vi "LVClasse_Phase GetStatisticDatas.vi"(0 "Phase in":refnum<class "Phase.lvclass">, 11 "error in (no error)":errorcluster) -> (4 "Phase out":refnum<class "Phase.lvclass">, 6 "StatisticsData":T1, 15 "error out":errorcluster)   [LabVIEW 2020, in "Phase.lvclass"]
doc: "Phase statistic data getter.\n\n--------------------------------------------------------------------------------\n\n<B>PhaseIn </B> : Phase object.\n<B>PhaseOut </B> : Phase object.\n<B>rms </B> : Phase root mean square deviation.\n<B>pv </B> : Phase peak to valley.\n<B>max </B> : Phase maximum.\n<B>min </B> : Phase minimum.\n<B>ErrorIn </B> : Error\n<B>ErrorOut </B> : Error\n\n--------------------------------------------------------------------------------"
uses:
  Phase.lvclass
  StatisticsData.ctl
  Phase.lvclass/Phase.ctl
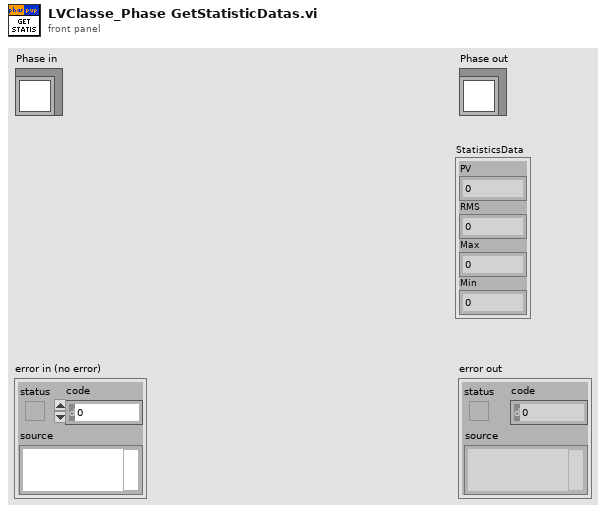
[diagram p1: front panel]
types:
  T1 = typedef "StatisticsData.ctl" = cluster{"PV":sgl, "RMS":dbl, "Max":sgl, "Min":sgl}
  T2 = cluster{"pv":dbl, "rms":dbl, "max":dbl, "min":dbl}
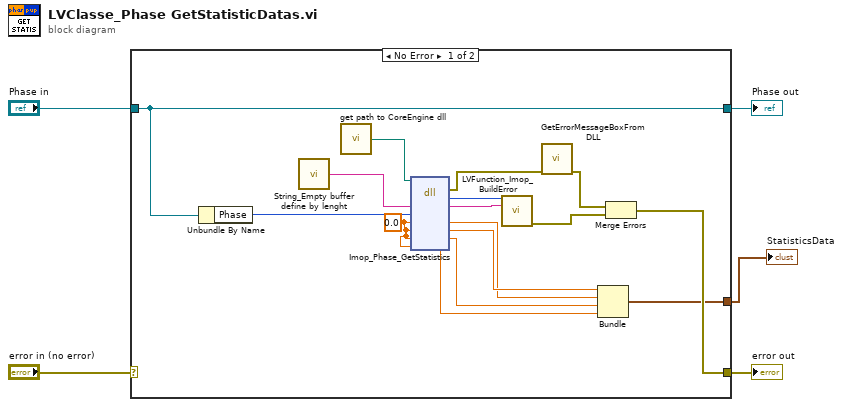
[diagram p0: block diagram]
diagram:
  n1 = case shown="No Error" "error in (no error)" {
    selector: "error in (no error)" -> [_ w23]
    tunnel: [w12 w23] -> w4
    tunnel: [w13 w22] -> w2
    tunnel: "Phase in" -> [w13 w22]
    tunnel: [w6 _] -> w1
    frame No Error {
      w11 = 0.0 ("rms")
      n2 = Unbundle By Name(w13) -> ("Phase"=w16:i32)
      n3 = call "String_Empty buffer define by lenght.vi"() -> ("Empty buffer"=w19:string)  [unwired: 1 in]
      n4 = call "get path to CoreEngine dll.vi"() -> ("path to c_interface_vc100.dll"=w18:path)  [unwired: 12 in, 3 out]
      n5 = dll-call lib="D:/soft/HASO_v3/SVN_trunk/ImOpCoreEngine4_LV2011/DLLs/c_interface_vc100.dll" fn="Imop_Phase_GetStatistics"(path in=w18, "message"=w19, "phase"=w16, "rms"=w11, "pv"=w11, "max"=w11, "min"=w11) -> (error out=w17:errorcluster, "return type"=w21:i32, "message"=w20:string, "rms"=w9:dbl, "pv"=w10:dbl, "max"=w8:dbl, "min"=w7:dbl)  [unwired: 3 in, 1 out]
      n6 = call "LVFunction_Imop_BuildError.vi"("code"=w21, "String to Prepend to source (\"\")"=w20) -> ("error out"=w14:errorcluster)  [unwired: 13 in]
      n7 = call "GetErrorMessageBoxFromDLL.vi"("error IN"=w17) -> ("error OUT"=w15:errorcluster)  [unwired: 10 in]
      n8 = Bundle("pv"=w10, "rms"=w9, "max"=w8, "min"=w7) -> (w6:T2)  [unwired: 1 in]
      n9 = Merge Errors(w15, w14) -> (w12:errorcluster)
    }
    frame Error {
    }
  }
  "error out" <- w4
  "Phase out" <- w2
  "StatisticsData" <- w1
